vi "Read Message.vi"(8 "error in (no error)":errorcluster, 11 "Control Box in":refnum<class "Control Box.lvclass">) -> (0 "error out":errorcluster, 1 "Remaining Channels":T1[](array[typedef]), 2 "Control Board":T1, 3 "Control Box out":refnum<class "Control Box.lvclass">)   [LabVIEW 2018, in "Control Box.lvlib" / "Control Box.lvclass"]
uses:
  Control Box.lvclass
  Custom Controls/Channel Status.ctl
  Control Box.lvlib
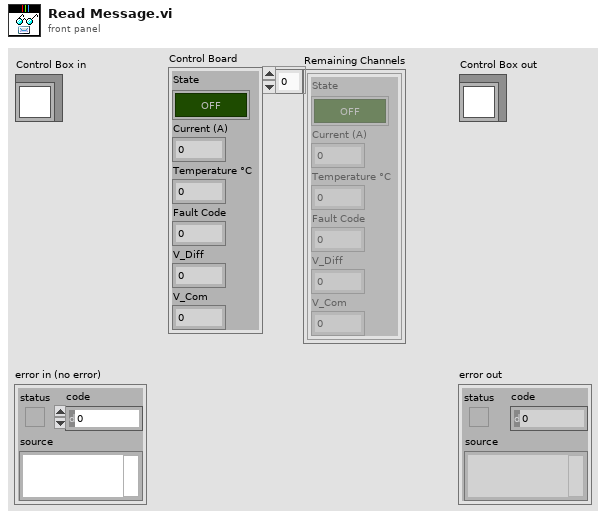
[diagram p1: front panel]
types:
  T1 = typedef "Control Box.lvlib/Channel Status.ctl" = cluster{"State":bool, "Current (A)":dbl, "Temperature °C":dbl, "Fault Code":u8, "V_Diff":dbl, "V_Com":dbl}
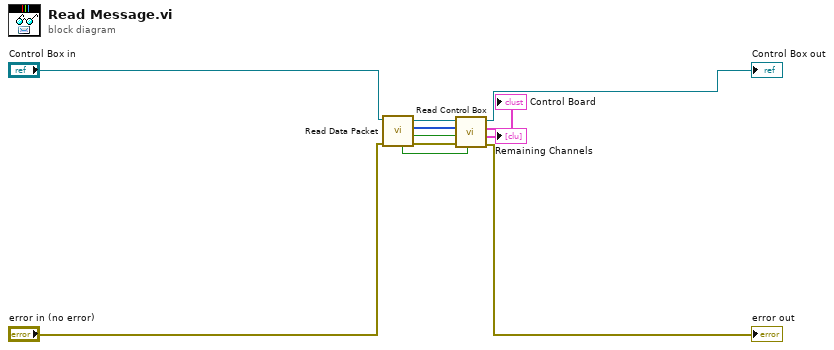
[diagram p0: block diagram]
diagram:
  n1 = call "Read Data Packet.vi"("error in (no error)"="error in (no error)", "Control Box in"="Control Box in") -> ("error out"=w4:errorcluster, "Bad Packet?"=w5:bool, "Raw Data"=w6:u8[], "Control Box out"=w7:refnum<class "Control Box.lvclass">, "Timeout?"=w3:bool)  [unwired: 5 in]
  n2 = call "Read Control Box.vi"("Timeout?"=w3, "error in (no error)"=w4, "Bad Packet?"=w5, "Raw Data"=w6, "Control Box in"=w7) -> ("error out"=→"error out":errorcluster, "Remaining Channels"=→"Remaining Channels":T1[], "Control Board"=→"Control Board":T1, "Control Box out"=→"Control Box out":refnum<class "Control Box.lvclass">)  [unwired: 3 in]
